vi "Shooting Method.vi"() -> ()   [LabVIEW 2023]
doc: "Solves a second-order differential equation using the shooting method."
uses:
  <vilib>/gmath/NI_Gmath.lvlib
panel:
  in  "Stop":bool
  out "XY Graph":T1(graph)
  out "x(1)-x1":dbl=-0.0036301982160208413 format="%0.2f"
  in  "y(0)":dbl(slide)=-0.114 scale=-0.2..0.2
  in  "x1":dbl=-0.1
  in  "x0":dbl
  in  "f(x,y,t)":string="sin(4*pi(1)*t)-100*(x*y)"
  # "Overview: Demonstrates the use of the ODE Runge Kutta 4th Order VI to solve the boundary value problem of a second order ODE by shooting method.\nRequirements: LabVIEW Full Development System\nInstructions:\n1. Run the VI.\n2. Modify the x0, x1, and y(0) values and observe the effects on the XY Graph, and the x(1)-x1 value.\n3. Click Stop to stop the VI."
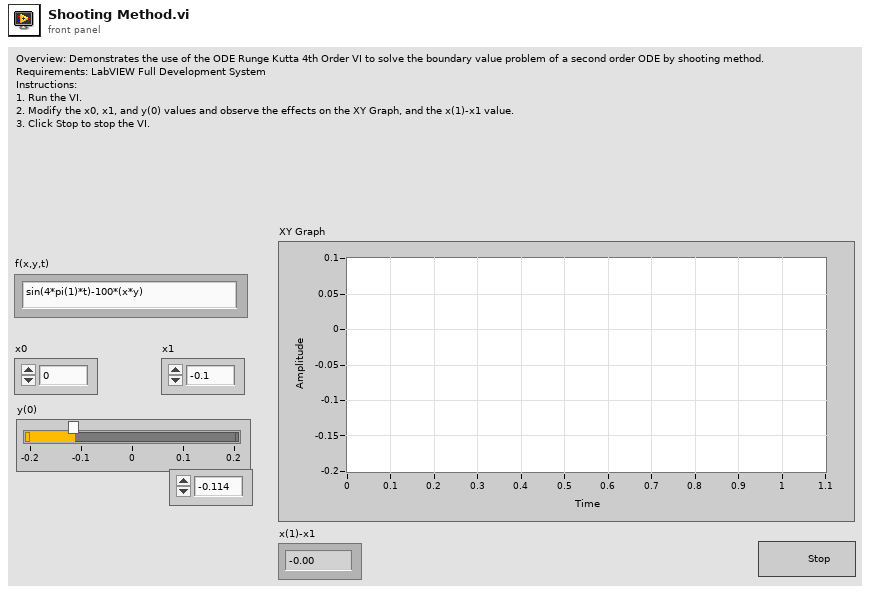
[diagram p1: front panel]
types:
  T1 = cluster{"Times":dbl[], "X Values (solution)":dbl[]}[]
  T2 = cluster{"Times":dbl[], "X Values (solution)":dbl[]}
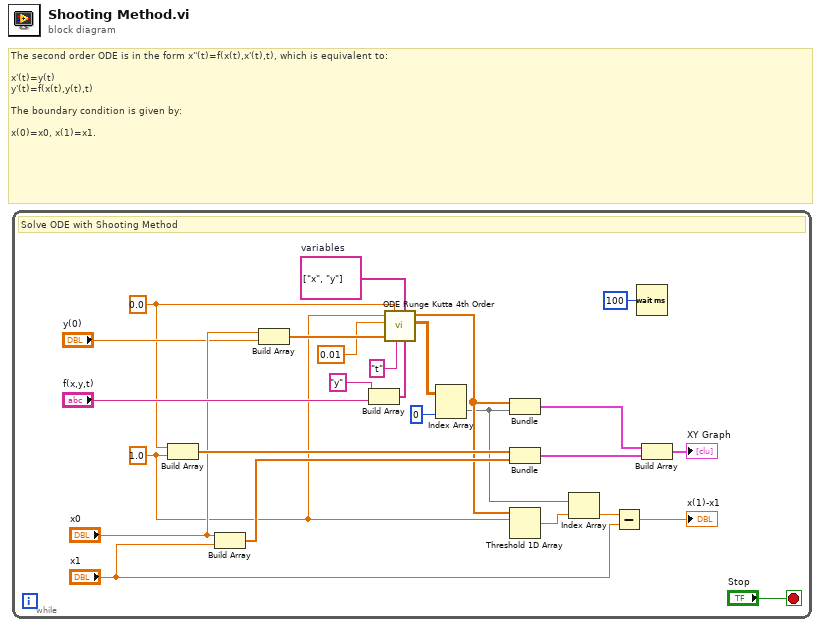
[diagram p0: block diagram]
diagram:
  # "The second order ODE is in the form x''(t)=f(x(t),x'(t),t), which is equivalent to:\n\nx'(t)=y(t)\ny'(t)=f(x(t),y(t),t)\n\nThe boundary condition is given by:\n\nx(0)=x0, x(1)=x1."
  n1 = while {
    stop <- "Stop" stop-if-true
    w3 = string[] ["x", "y"]  # variables
    w6 = 1.0
    w7 = 0.0
    # "Solve ODE with Shooting Method"
    n2 = Build Array(w7, w6) -> (w26:dbl[])
    n3 = Build Array("x0", "x1") -> (w25:dbl[])
    n4 = Build Array("x0", "y(0)") -> (w20:dbl[])
    n5 = Build Array("y", "f(x,y,t)") -> (w22:string[])
    n6 = call <vilib>:"ODE Runge Kutta 4th Order.vi"("time end"=w6, "time start"=w7, "h (step rate)"=0.01, "X0"=w20, "time"="t", "X (name of variables)"=w3, "F(X,t) (right sides of the ODE\nas functions of X and t)"=w22) -> ("Times"=w11:dbl[], "X Values (solution)"=w19:dbl[][])  [unwired: 2 out]
    n7 = Index Array(array=w19, index (col)=0) -> (element=w8:dbl[])  [unwired: 1 in]
    n8 = Bundle("Times"=w11, "X Values (solution)"=w8) -> (w18:T2)  [unwired: 1 in]
    n9 = Bundle(w26, w25) -> (w17:cluster{dbl[], dbl[]})  [unwired: 1 in]
    n10 = Threshold 1D Array(2:w6, 3:w11) -> (0:w13:dbl)  [unwired: 1 in]
    n11 = Index Array(array=w8, index=w13) -> (element=w10:dbl)
    n12 = Subtract(x=w10, y="x1") -> (x-y=→"x(1)-x1":dbl)
    n13 = Wait (ms)(milliseconds to wait=u32 100) -> ()  [unwired: 1 out]
    n14 = Build Array(w18, w17) -> (→"XY Graph":T1)
  }
